vi "HDI Pad Group Deviation.vi"() -> ()   [LabVIEW 2011]
uses:
  Shared Components/Gantry Class/Gantry Class.lvclass
  Shared Components/WorkTable Class/WorkTable Class.lvclass
  Shared Components/CameraTool Class/CameraTool Class.lvclass
  Shared Components/Vec3d Class/Vec3d Class.lvclass
panel:
  in  "Tab Control":enum32{"Control", "Results"}(tab)
  out "preview":T1(plugin-control)
  in  "Config Folder":path=path "C:/Users/Husker/Desktop/gantry/Config"
  in  "capture pos":bool
  out "results":string
  out "error out":errorcluster
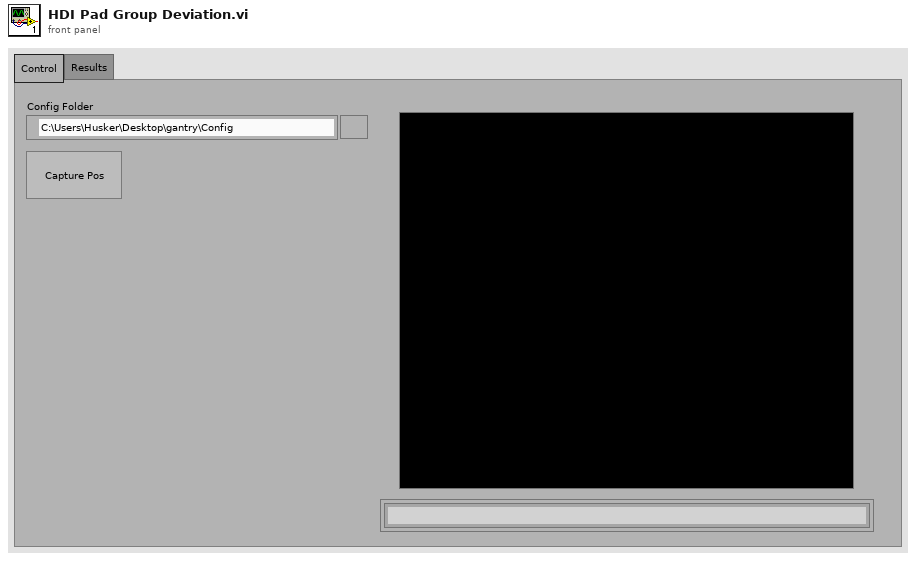
[diagram p1: front panel]
types:
  T1 = typedef "IMAQ Image.ctl" = refnum<image>
  T2 = typedef "Worktable_Module Slot.ctl" = cluster{"Slot State":enum16{"Empty", "Unglued", "Stamped", "PartOnTop", "Weighted", "Unpotted", "Potted"}, "BBM Type":enum16{"None", "BBM", "GlassSlide"}, "HDI Type":enum16{"None", "HDI", "Polyimide"}, "Vacuum Channel":u8, "Location/Orientation BBM":T3, "Location/Orientation HDI":T3, "S/N":string}
  T3 = typedef "Position_Orientation.ctl" = cluster{"Center":refnum<class "Vec3d Class.lvclass">, "Orientation":refnum<class "Orient3d Class.lvclass">}
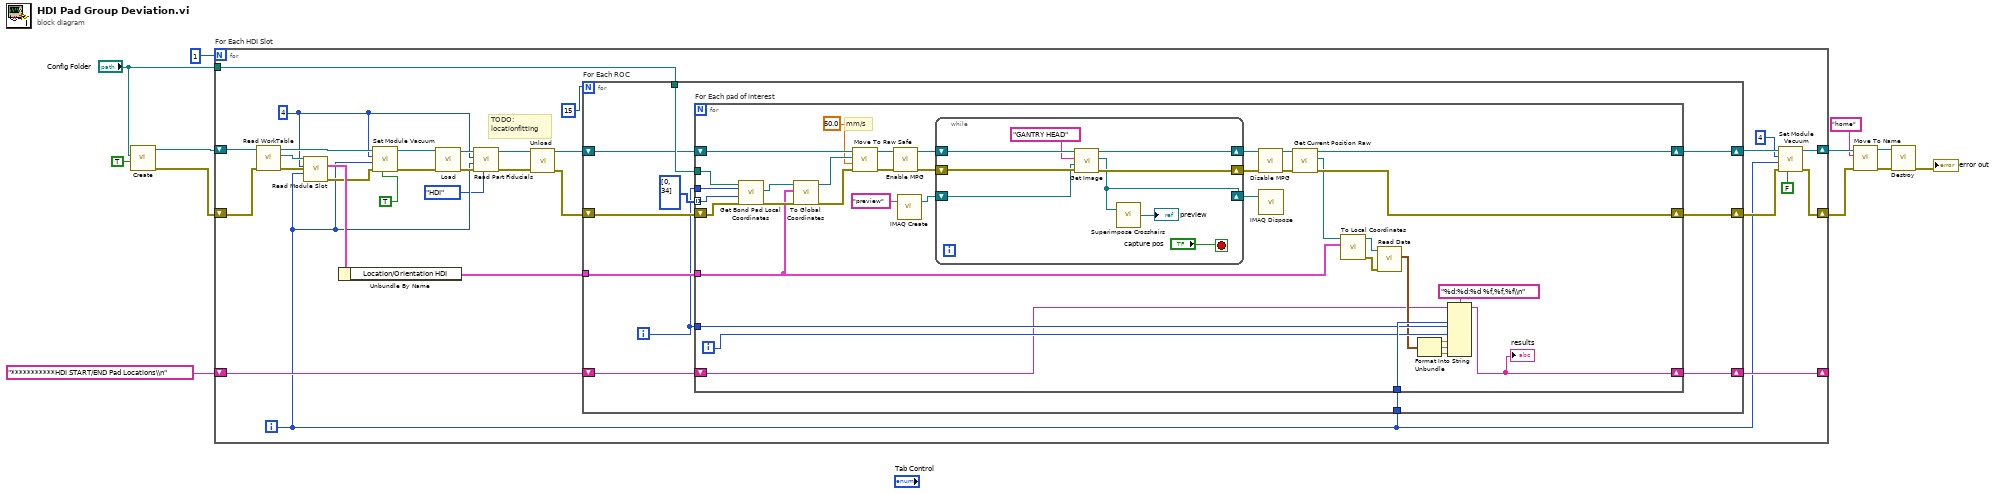
[diagram p0: block diagram]
diagram:
  n1 = call "Create.vi"("HOME?"=TRUE, "Config Folder"="Config Folder") -> ("error out"=w1:errorcluster, "Gantry out"=w2:refnum<class "Gantry Class.lvclass">)  [unwired: 8 in]
  n2 = for "For Each HDI Slot" {
    N: 1 -> [_]
    tunnel: "Config Folder" -> [w41]
    shift-right: [w27] -> w9
    shift-left: w2 -> [w40]
    shift-right: [w33] -> _
    shift-left: "***********HDI START/END Pad Locations\\n" ("results") -> [w34]
    shift-right: [w25] -> w4
    shift-left: w1 -> [w35]
    i -> [w16]
    w15 = 4 ("chuck")
    # "TODO:\nlocationfitting"
    n3 = call-dynamic "Read WorkTable.vi"("error in"=w35, "Gantry Class in"=w40) -> ("error out"=w39:errorcluster, "WorkTable Class.lvclass"=w38:refnum<class "WorkTable Class.lvclass">, "Gantry Class out"=w32:refnum<class "Gantry Class.lvclass">)  [unwired: 7 in]
    n4 = call-dynamic "Read Module Slot.vi"("error in"=w39, "slot"=w16, "chuck"=w15, "WorkTable in"=w38) -> ("error out"=w31:errorcluster, "Module Slot"=w37:T2)  [unwired: 5 in, 1 out]
    n5 = Unbundle By Name(w37) -> ("Location/Orientation HDI"=w36:T3)
    n6 = call-dynamic "Set Module Vacuum.vi"("On/Off"=TRUE, "error in"=w31, "Slot Number"=w16, "Chuck Number"=w15, "Gantry in"=w32) -> ("error out"=w18:errorcluster, "Gantry out"=w20:refnum<class "Gantry Class.lvclass">)  [unwired: 5 in]
    n7 = call "Load.vi"("error in"=w18, "Gantry In"=w20) -> ("error out"=w24:errorcluster, "CameraTool out"=w23:refnum<class "CameraTool Class.lvclass">)  [unwired: 8 in]
    n8 = call-dynamic "Read Part Fiducials.vi"("Part Type"=enum16{"HDI", "BBM", "HDI-on-BBM"}."HDI", "error in"=w24, "Slot"=w16, "Chuck"=w15, "CameraTool in"=w23) -> ("error out"=w22:errorcluster, "CameraTool out"=w21:refnum<class "CameraTool Class.lvclass">)  [unwired: 4 in, 1 out]
    n9 = call "Unload.vi"("error in"=w22, "CameraTool in"=w21) -> ("error out"=w17:errorcluster, "Gantry out"=w19:refnum<class "Gantry Class.lvclass">)  [unwired: 8 in]
    n10 = for "For Each ROC" {
      N: 15 -> [_]
      tunnel: w41 -> [w53]
      tunnel: w36 -> [w52]
      shift-right: [w48] -> w28
      shift-left: w19 -> [w50]
      tunnel: w16 -> [w47]
      shift-right: [w44] -> w33
      shift-left: w34 -> [w45]
      shift-right: [w43] -> w26
      shift-left: w17 -> [w51]
      i -> [w46]
      n11 = for "For Each pad of interest" {
        tunnel: w53 -> [w90]
        tunnel: w52 -> [w71]
        shift-right: [w72] -> w43
        shift-left: w51 -> [w87]
        tunnel: w46 -> [w83]
        tunnel: i32[] [0, 34] -> [w82] mode=indexing
        shift-right: [w73] -> w48
        shift-left: w50 -> [w86]
        tunnel: w47 -> [w66]
        tunnel: w46 -> [w65]
        shift-right: [w58] -> w44
        shift-left: w45 -> [w59]
        i -> [w64]
        # "mm/s"
        n12 = call "Get Bond Pad Local Coordinates.vi"("error in"=w87, "ROC Pad Number"=w82, "ROC"=w83, "Config Location"=w90) -> ("error out"=w88:errorcluster, "Pad Local Coordinates"=w89:refnum<class "Vec3d Class.lvclass">)  [unwired: 6 in]
        n13 = call "To Global Coordinates.vi"("error in"=w88, "Center/Orientation"=w71, "Local Coordinates"=w89) -> ("error out"=w84:errorcluster, "Global Coordinates"=w85:refnum<class "Vec3d Class.lvclass">)  [unwired: 7 in]
        n14 = call-dynamic "Move To Raw Safe.vi"("error in"=w84, "Speed"=50.0, "Destination"=w85, "Gantry in"=w86) -> ("error out"=w80:errorcluster, "Gantry out"=w81:refnum<class "Gantry Class.lvclass">)  [unwired: 6 in]
        n15 = call-dynamic "Enable MPG.vi"("error in (no error)"=w80, "Gantry Class in"=w81) -> ("error out"=w78:errorcluster, "Gantry Class out"=w79:refnum<class "Gantry Class.lvclass">)  [unwired: 8 in]
        n16 = call "IMAQ Create"("Image Name"="preview") -> ("New Image"=w56:T1)  [unwired: 4 in, 1 out]
        n17 = while {
          shift-right: [w95] -> w77
          shift-left: w78 -> [w98]
          shift-right: [w96] -> w76
          shift-left: w79 -> [w99]
          shift-right: [w91] -> w55
          shift-left: w56 -> [w93]
          stop <- "capture pos" stop-if-true
          n18 = call-dynamic "Get Image.vi"("error in"=w98, "Image In"=w93, "Camera Name"="GANTRY HEAD", "Gantry in"=w99) -> ("error out"=w95:errorcluster, "Image Out"=w91:T1, "Gantry out"=w96:refnum<class "Gantry Class.lvclass">)  [unwired: 4 in, 1 out]
          n19 = call "Superimpose Crosshairs.vi"("Refnum in"=w91) -> ("Refnum out"=→"preview":T1)  [unwired: 1 in]
        }
        n20 = call-dynamic "Disable MPG.vi"("error in"=w77, "Gantry in"=w76) -> ("error out"=w75:errorcluster, "Gantry out"=w74:refnum<class "Gantry Class.lvclass">)  [unwired: 8 in]
        n21 = call "IMAQ Dispose"("Image"=w55) -> ()  [unwired: 5 in, 1 out]
        n22 = call-dynamic "Get Current Position Raw.vi"("error in (no error)"=w75, "Gantry Class in"=w74) -> ("error out"=w72:errorcluster, "Vec3d Class out"=w70:refnum<class "Vec3d Class.lvclass">, "Gantry Class out"=w73:refnum<class "Gantry Class.lvclass">)  [unwired: 7 in]
        n23 = call "To Local Coordinates.vi"("Center/Orientation"=w71, "Global Coordinates"=w70) -> ("error out"=w69:errorcluster, "Local Coordinates"=w68:refnum<class "Vec3d Class.lvclass">)  [unwired: 8 in]
        n24 = call-dynamic "Read Data.vi"("error in (no error)"=w69, "Vec3d Class in"=w68) -> ("Data"=w63:cluster{"X":dbl, "Y":dbl, "Z":dbl})  [unwired: 7 in, 2 out]
        n25 = Unbundle(w63) -> ("X"=w62:dbl, "Y"=w61:dbl, "Z"=w60:dbl)
        n26 = Format Into String(format string="%d:%d:%d %f,%f,%f\\n", initial string=w59, w66, w65, w64, w62, w61, w60) -> (resulting string=w58:string)  [unwired: 1 in, 1 out]
        "results" <- w58
      }
    }
    n27 = call-dynamic "Set Module Vacuum.vi"("On/Off"=FALSE, "error in"=w26, "Slot Number"=w16, "Chuck Number"=4, "Gantry in"=w28) -> ("error out"=w25:errorcluster, "Gantry out"=w27:refnum<class "Gantry Class.lvclass">)  [unwired: 5 in]
  }
  n28 = call-dynamic "Move To Name.vi"("error in"=w4, "Destination Name"="home", "Gantry in"=w9) -> ("error out"=w5:errorcluster, "Gantry out"=w6:refnum<class "Gantry Class.lvclass">)  [unwired: 7 in]
  n29 = call "Destroy.vi"("error in"=w5, "Gantry Class in"=w6) -> ("error out"=→"error out":errorcluster)  [unwired: 9 in]
